vi "User Access Level FGV Unit Test.vi"() -> ()   [LabVIEW 2012]
uses:
  User Level FGV/User Level Cmd.ctl
panel:
  in  "Test Access Level":bool
  out "Error Out":errorcluster
  in  "Error In":errorcluster
  in  "Current User":string
  in  "Set Current User":bool
  in  "stop":bool
  # "1.  Set access level for current user."
  # "2.  Test access level by verifying the appropriate dialog message."
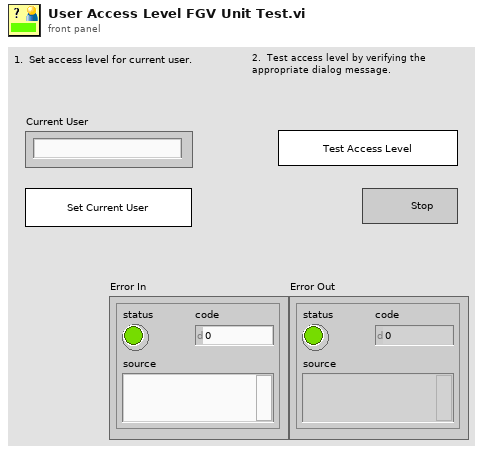
[diagram p1: front panel]
types:
  T1 = typedef "User Level Cmd.ctl" = enum16{"Read User Access Level File", "Set Current User", "Get User Access Level"}
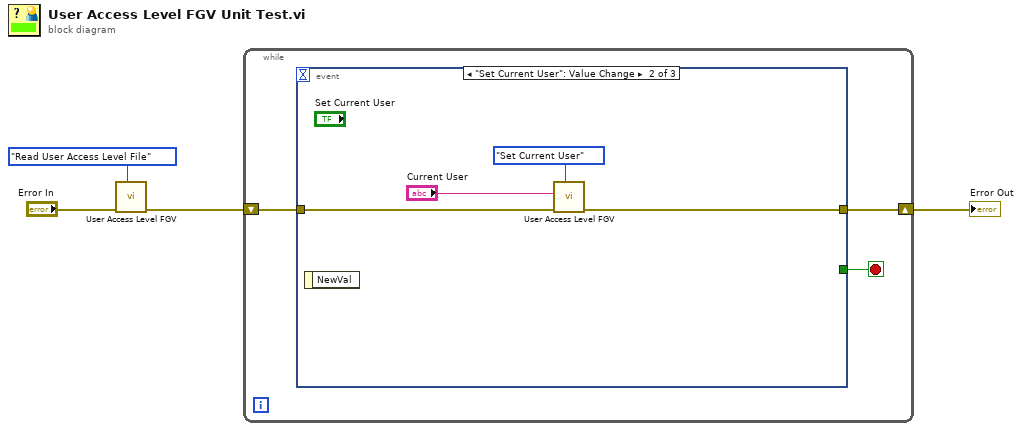
[diagram p0: block diagram]
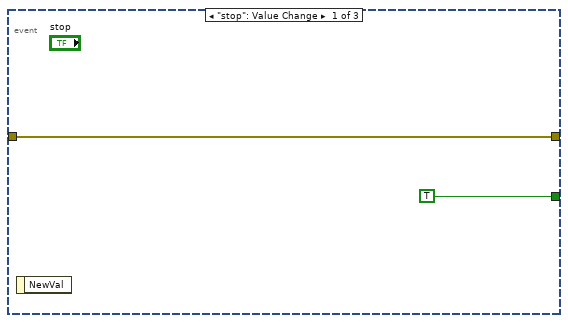
[diagram p2: hidden frame]
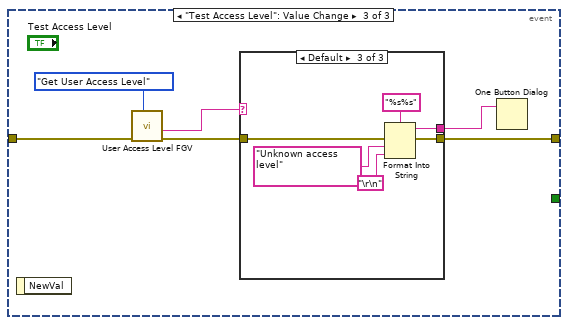
[diagram p3: hidden frame]
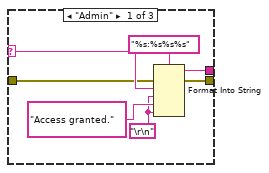
[diagram p4: hidden frame]
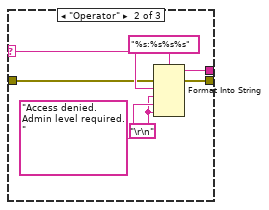
[diagram p5: hidden frame]
diagram:
  n1 = call "User Access Level FGV.vi"("User Level Cmd"=User_Level_Cmd."Read User Access Level File", "Error In"="Error In") -> ("Error Out"=w4:errorcluster)  [unwired: 8 in, 1 out]
  n2 = while {
    shift-right: [w5] -> w1
    shift-left: w4 -> [w6]
    stop <- w7 stop-if-true
    n3 = event shown="[1] \"Set Current User\": Value Change" {
      selector: _ -> [_ _ _]
      dyn-events: _ -> [_ _ _]
      timeout: _ -> [_ _ _]
      tunnel: [TRUE ("stop") _ _] -> w7
      tunnel: w6 -> [w8 w12 w18]
      tunnel: [w8 w10 w17] -> w5
      event "stop": Value Change {
        n4 = event-data() -> ()  [unwired: 1 in, 1 out]
      }
      event "Set Current User": Value Change {
        n5 = event-data() -> ()  [unwired: 1 in, 1 out]
        n6 = call "User Access Level FGV.vi"("User Level Cmd"=User_Level_Cmd."Set Current User", "Error In"=w12, "User Name"="Current User") -> ("Error Out"=w10:errorcluster)  [unwired: 7 in, 1 out]
      }
      event "Test Access Level": Value Change {
        n7 = event-data() -> ()  [unwired: 1 in, 1 out]
        n8 = call "User Access Level FGV.vi"("User Level Cmd"=User_Level_Cmd."Get User Access Level", "Error In"=w18) -> ("Error Out"=w16:errorcluster, "User Level"=w15:string)  [unwired: 8 in]
        n9 = case shown="Default" w15 {
          selector: w15 -> [w26 w33 _]
          tunnel: [w24 w31 w38] -> w17
          tunnel: w16 -> [w25 w32 w39]
          tunnel: [w20 w27 w36] -> w14
          frame "Admin" {
            w22 = "\r\n"
            n10 = Format Into String(format string="%s:%s%s%s", error in=w25, w26, w22, "Access granted." ("message"), w22) -> (resulting string=w20:string, error out=w24:errorcluster)  [unwired: 1 in]
          }
          frame "Operator" {
            w29 = "\r\n"
            n11 = Format Into String(format string="%s:%s%s%s", error in=w32, w33, w29, "Access denied.  Admin level required." ("message"), w29) -> (resulting string=w27:string, error out=w31:errorcluster)  [unwired: 1 in]
          }
          frame Default {
            n12 = Format Into String(format string="%s%s", error in=w39, "Unknown access level" ("message"), "\r\n") -> (resulting string=w36:string, error out=w38:errorcluster)  [unwired: 1 in]
          }
        }
        n13 = One Button Dialog(message=w14) -> ()  [unwired: 1 in, 1 out]
      }
    }
  }
  "Error Out" <- w1
